vi "StateLimeLight.vi"(1 "Master State":string) -> ()   [LabVIEW 2019]
doc: "This VI manages the LimeLight pipelines and LimeLight targeting LED mode."
uses:
  <vilib>/Rock Robotics/WPI/DriverStation/WPI_DriverStationRobotMode2.ctl
  dsdata.vi
  sensors.vi
  outputs.vi
  dscommands.vi
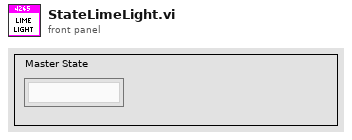
[diagram p1: front panel]
types:
  T1 = typedef "WPI_DriverStationRobotMode2.ctl" = enum16{"Autonomous Disabled", "Autonomous Enabled", "Teleop Disabled", "Teleop Enabled", "Disconnected", "Finish", "Test Disabled", "Test Enabled", "Emergency Stopped"}
  T2 = enum16{"Boot Up", "Camera Override", "Power Port", "Ball Tracking"}
  T3 = enum16{"Driver Control", "Auto Targeting", "Feeder Station"}
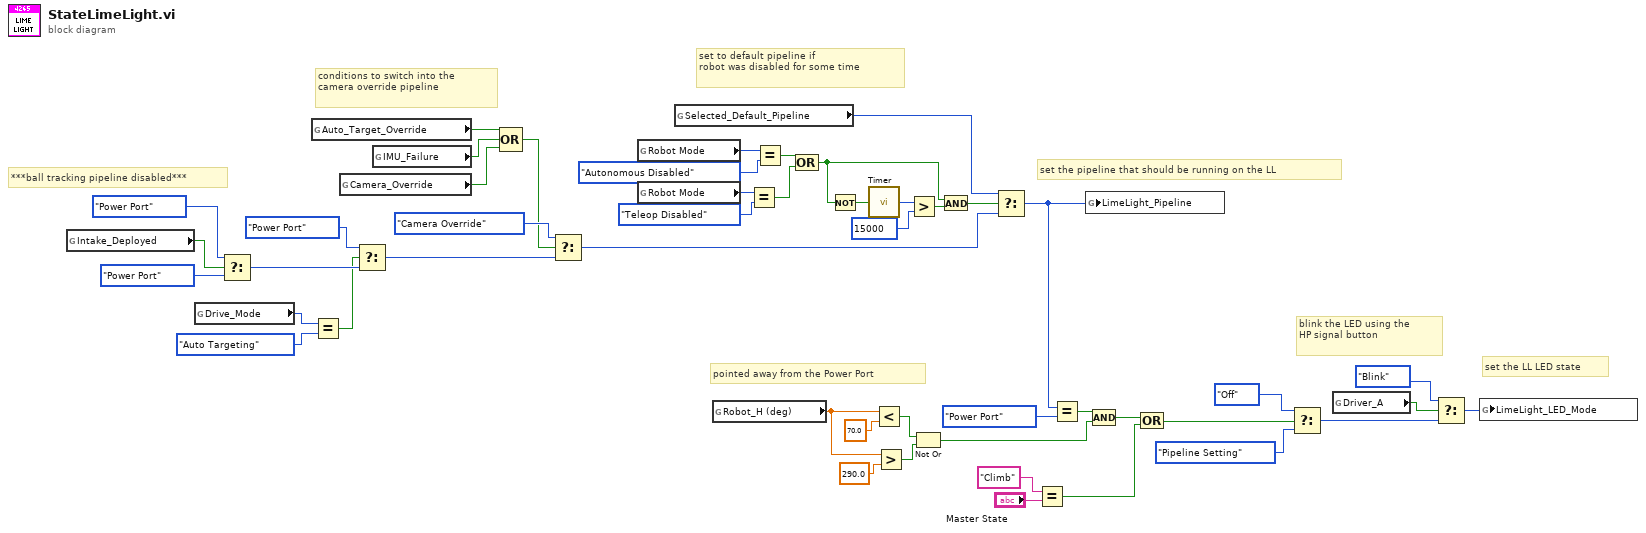
[diagram p0: block diagram]
diagram:
  # "***ball tracking pipeline disabled***"
  # "set to default pipeline if \nrobot was disabled for some time"
  # "set the LL LED state"
  # "pointed away from the Power Port"
  # "conditions to switch into the \ncamera override pipeline"
  # "set the pipeline that should be running on the LL"
  # "blink the LED using the\nHP signal button"
  n1 = global read "outputs.vi" "Intake_Deployed"() -> (w44:bool)
  n2 = global read "outputs.vi" "Drive_Mode"() -> (w26:T3)
  n3 = Select(t=T2."Power Port", s=w44, f=T2."Power Port") -> (s? t:f=w23:T2)
  n4 = global read "dsdata.vi" "Auto_Target_Override"() -> (w48:bool)
  n5 = Equal?(x=w26, y=T3."Auto Targeting") -> (x = y?=w22:bool)
  n6 = global read "dsdata.vi" "Camera_Override"() -> (w46:bool)
  n7 = Select(t=T2."Power Port", s=w22, f=w23) -> (s? t:f=w21:T2)
  n8 = global read "sensors.vi" "IMU_Failure"() -> (w47:bool)
  n9 = Compound Arithmetic op=OR(w48, w47, w46) -> (w42:bool)
  n10 = Select(t=T2."Camera Override", s=w42, f=w21) -> (s? t:f=w14:T2)
  n11 = global read "dsdata.vi" "Robot Mode"() -> (w20:T1)
  n12 = global read "dsdata.vi" "Robot Mode"() -> (w17:T1)
  n13 = global read "dsdata.vi" "Selected_Default_Pipeline"() -> (w12:T2)
  n14 = global read "sensors.vi" "Robot_H (deg)"() -> (w31:dbl)
  n15 = Equal?(x=w17, y=WPI_DriverStationRobotMode2."Teleop Disabled") -> (x = y?=w15:bool)
  n16 = Equal?(x=w20, y=WPI_DriverStationRobotMode2."Autonomous Disabled") -> (x = y?=w18:bool)
  n17 = Compound Arithmetic op=OR(w18, w15) -> (w10:bool)
  n18 = Not(x=w10) -> (.not. x?=w9:bool)
  n19 = call "Timer.vi"("Reset Timer"=w9) -> ("Time (ms)"=w7:u32)
  n20 = Less?(x=w31, y=70.0) -> (x < y?=w32:bool)
  n21 = Greater?(x=w31, y=290.0) -> (0:w33:bool)
  n22 = Greater?(x=w7, y=u32 15000 ("x")) -> (0:w13:bool)
  n23 = Not Or(1:w33, 2:w32) -> (0:w28:bool)
  n24 = And(x=w10, y=w13) -> (x .and. y?=w11:bool)
  n25 = Select(t=w12, s=w11, f=w14) -> (s? t:f=w8:T2)
  n26 = Equal?(x="Climb", y="Master State") -> (x = y?=w1:bool)
  n27 = Equal?(x=w8, y=T2."Power Port") -> (x = y?=w30:bool)
  n28 = global write "outputs.vi" "LimeLight_Pipeline"(w8) -> ()
  n29 = Compound Arithmetic op=AND(w30, w28) -> (w5:bool)
  n30 = Compound Arithmetic op=OR(w5, w1) -> (w4:bool)
  n31 = Select(t=enum16{"Pipeline Setting", "Off", "Blink", "On"}."Off", s=w4, f=enum16{"Pipeline Setting", "Off", "Blink", "On"}."Pipeline Setting") -> (s? t:f=w37:enum16{"Pipeline Setting", "Off", "Blink", "On"})
  n32 = global read "dscommands.vi" "Driver_A"() -> (w40:bool)
  n33 = Select(t=enum16{"Pipeline Setting", "Off", "Blink", "On"}."Blink", s=w40, f=w37) -> (s? t:f=w36:enum16{"Pipeline Setting", "Off", "Blink", "On"})
  n34 = global write "outputs.vi" "LimeLight_LED_Mode"(w36) -> ()
